vi "ChiSquareCalculation.vi"(2 "Extinction ExtinctionUncertainity Size parameter and Number ofS sizes 2":T1={"PAS amplitude"=[], "PAS amp Uncertainty"=[], "Size parameters"=[], "Number ofSizes"=0.0, "GeometricCrossSection"=[], "Wave Length"=0.0, "SMPS Sizes"=[], "Concentration"=[], "Double Charge Correction"=FALSE, "Extincation Factor"=1.0, "Diameter Factor"=1.0, "Diameter Offset"=0.0, "Extinction Factor Flag"=FALSE, "Diameter Factor Flag"=FALSE, "Diameter Offset Flag"=FALSE, "Sizes"=[], "ExtinctionOrAbsorptionOrScattering"=0, "Concentration(#/cc)"=[]} {"ExtinctionOrAbsorptionOrScattering" scale=0.0..2.0}, 3 "refractive index, imaginary":dbl=0.037 format="%.5f", 4 "refractive index, real":dbl=1.567 format="%.5f") -> (0 "Normalized Residuals":dbl[](array[numeric])=[0.11611698626140751, -0.00782281527933284, -0.39724759167122026, -0.05829577642327765, 0.5102944282210912], 1 "Chi Squared":dbl=0.43514880104819414)   [LabVIEW 2013]
uses:
  BaesDataTypeDefinition.ctl
panel:
  out "Normalized Residuals 2":dbl[](array[numeric])=[0.11611698626140751, -0.00782281527933284, -0.39724759167122026, -0.05829577642327765, 0.5102944282210912]
  out "Absorption Coef Predicted Mie":dbl[](array[numeric])
  out "Expected Value For R and I refractive Index":sgl[](array[numeric])=[1.8559851e-09, 2.336765e-09, 2.8534894e-09, 3.365495e-09, 4.0278967e-09]
  # "Mie scattering demo program, August 2005, by Martin Fierz (martin@fierz.ch)\n\nThis VI demonstrates the usage of mie2.dll; a dynamic-link-library which you can call in your LabView program.\nThe demo lets you select the refractive index of a sphere, and the size parameter and computes total scattering,\ntotal extinction and angular distribution of the scattered light for p-, s- and unpolarized light.\nMie2.dll uses the Bohren-Huffman Mie code."
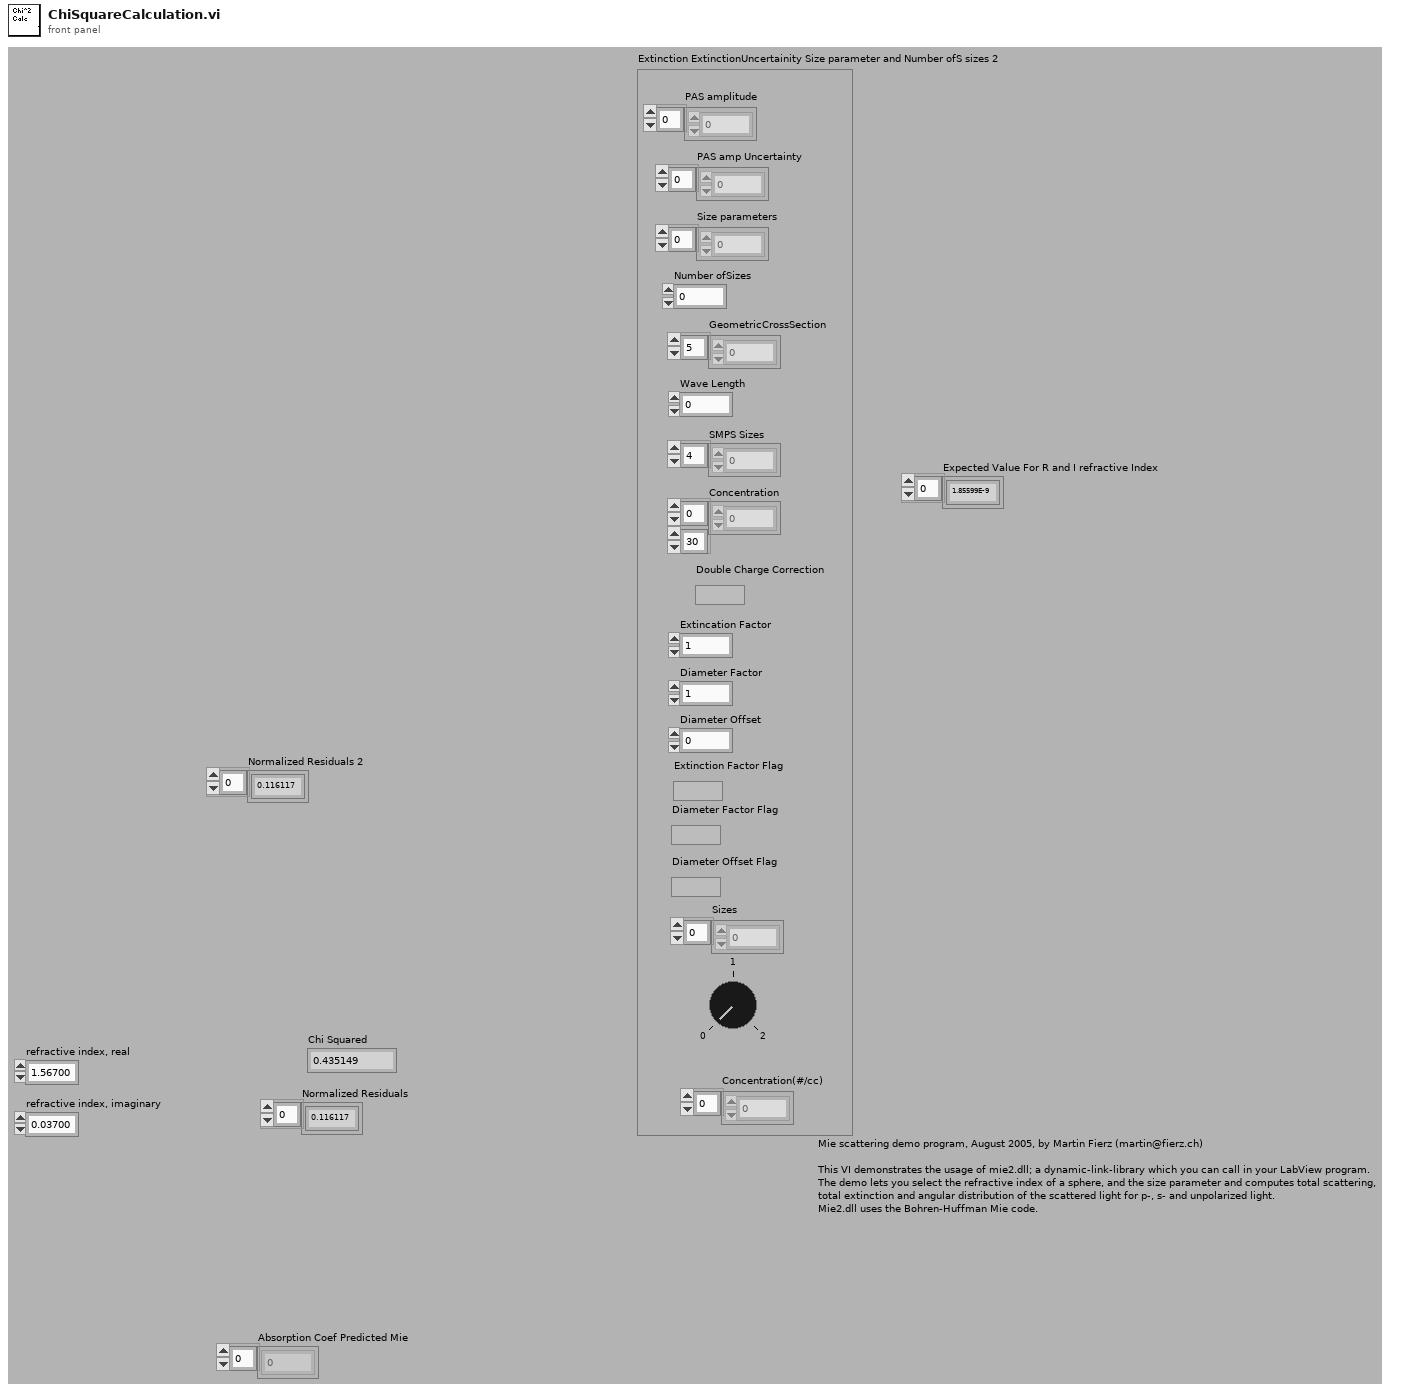
[diagram p1: front panel]
types:
  T1 = typedef "BaesDataTypeDefinition.ctl" = cluster{"PAS amplitude":dbl[], "PAS amp Uncertainty":dbl[], "Size parameters":dbl[], "Number ofSizes":dbl, "GeometricCrossSection":dbl[], "Wave Length":dbl, "SMPS Sizes":dbl[], "Concentration":dbl[][], "Double Charge Correction":bool, "Extincation Factor":dbl, "Diameter Factor":dbl, "Diameter Offset":dbl, "Extinction Factor Flag":bool, "Diameter Factor Flag":bool, "Diameter Offset Flag":bool, "Sizes":dbl[], "ExtinctionOrAbsorptionOrScattering":i8, "Concentration(#/cc)":dbl[]}
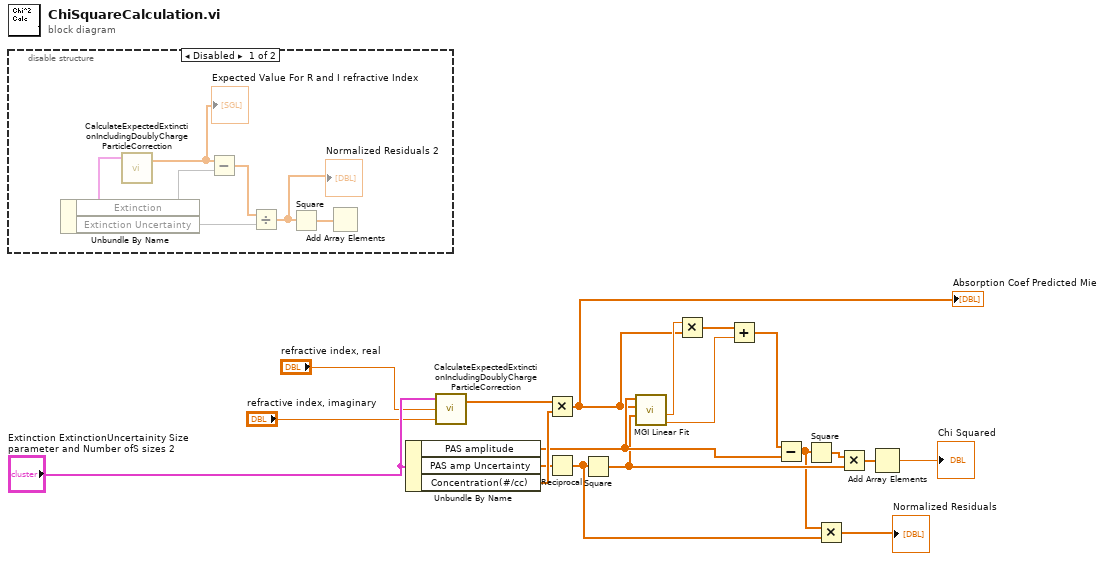
[diagram p0: block diagram]
diagram:
  n1 = disable-structure shown="Disabled" {
    frame Disabled {
      n2 = Unbundle By Name() -> (w21:T1, "Extinction"=w25, "Extinction Uncertainty"=w24)
      n3 = call "CalculateExpectedExtinctionIncludingDoublyChargeParticleCorrection.vi"("Extinction ExtinctionUncertainity Size parameter and Number ofS sizes"=w21) -> ("Expected Extinction/Absorption Cross Section"=w22:sgl[], "refractive index, real"=w23:sgl)  [unwired: 1 in, 1 out]
      "Expected Value For R and I refractive Index" <- w22
      n4 = Subtract(x=w22, y=w25) -> (x-y=w27:sgl[])
      n5 = Divide(x=w27, y=w24) -> (x/y=w20:sgl[])
      "Normalized Residuals 2" <- w20
      n6 = Square(x=w20) -> (x^2=w26:sgl[])
      n7 = Add Array Elements(numeric array=w26) -> ()  [unwired: 1 out]
    }
    frame Enabled {
    }
  }
  n8 = Unbundle By Name("Extinction ExtinctionUncertainity Size parameter and Number ofS sizes 2") -> ("PAS amplitude"=w11:dbl[], "PAS amp Uncertainty"=w14:dbl[], "Concentration(#/cc)"=w18:dbl[])
  n9 = call "CalculateExpectedExtinctionIncludingDoublyChargeParticleCorrection.vi"("refractive index, imaginary"="refractive index, imaginary", "refractive index, real"="refractive index, real", "Extinction ExtinctionUncertainity Size parameter and Number ofS sizes"="Extinction ExtinctionUncertainity Size parameter and Number ofS sizes 2") -> ("Expected Extinction/Absorption Cross Section"=w19:sgl[])  [unwired: 1 out]
  n10 = Multiply(x=w19, y=w18) -> (x*y=w8:dbl[])
  "Absorption Coef Predicted Mie" <- w8
  n11 = Reciprocal(x=w14) -> (1/x=w2:dbl[])
  n12 = Square(x=w2) -> (x^2=w10:dbl[])
  n13 = call <userlib>:"MGI Linear Fit.vi"("Weights (equal)[]"=w10, "Xin[]"=w8, "Yin[]"=w11) -> ("Intercept"=w6:dbl, "Slope"=w9:dbl)  [unwired: 5 in, 2 out]
  n14 = Multiply(x=w9, y=w8) -> (x*y=w7:dbl[])
  n15 = Add(x=w7, y=w6) -> (x+y=w5:dbl[])
  n16 = Subtract(x=w5, y=w11) -> (x-y=w3:dbl[])
  n17 = Square(x=w3) -> (x^2=w13:dbl[])
  n18 = Multiply(x=w3, y=w2) -> (x*y=→"Normalized Residuals":dbl[])
  n19 = Multiply(x=w13, y=w10) -> (x*y=w12:dbl[])
  n20 = Add Array Elements(numeric array=w12) -> (sum=→"Chi Squared":dbl)
